vi "EOL Audit Display Data.vi"(7 "Check Position":T2, 8 "Check Noise Test":T2, 9 "Audit Motion Database Table":T3={"Motion"=enum."Glass Teach", "Actual Avg Current"=0.0, "Actual Runtime"=0.0, "Actual Speed"=0.0, "Current Data"=[], "Motion Data Limits"={"Power Supply Voltage"=0.0, "Min Avg Current"=0.0, "Max Avg Current"=0.0, "Min Run Time"=0.0, "Max Run Time"=0.0, "Min Speed"=0.0, "Max Speed"=0.0, "AP Data % of Threshold"=10.0, "Travel Distance"=0.0, "AP Data Type"=enum."91/61", "Check Current"=FALSE, "Check Run Time"=FALSE, "Check Speed"=FALSE, "Express Motion?"=FALSE, "Check Sound Test"=FALSE, "Check Position?"=FALSE, "Collect AP Data"=FALSE, "Inital Position"=0, "End Position"=0, "Goto Posiition"=0, "Max max Current"=0.0, "Min max Current"=0.0, "Check max Current"=FALSE, "Check Sound"=FALSE, "Min Sound (dB)"=0.0, "Max Sound (dB)"=0.0, "SW Mode"=enum."Hard Switch", "LIN Msg"={"ID"=0, "Msg"=[], "LDF"="EX1H"}}, "Switch 1 to 6"=[], "Actual PS Voltage"=0.0, "AP Data"=[], "Actual max Current"=0.0, "Actual Noise (dB)"=0.0} {"Motion Data Limits"."LIN Msg"."Msg" format="%02x"; "Motion Data Limits"."LIN Msg"."ID" format="%02x"}) -> (2 "Limits Data":T1 {"Speed" format="%.2g"; "Run Time" format="%.2g"; "Avg Current" format="%.2g"}, 3 "Actual Data":T1 {"Speed" format="%.2g"; "Run Time" format="%.2g"; "Avg Current" format="%.2g"})   [LabVIEW 2018]
uses:
  02.Type Def's/EOL Motion Database Table.ctl
  02.Type Def's/All Motions.ctl
  05.UserVI's/type defs/17x Audit Motion Data Seq Control.ctl
  05.UserVI's/type defs/17x AP Data Type.ctl
  02.Type Def's/Pass Fail Control.ctl
  02.Type Def's/Screen Motion Data.ctl
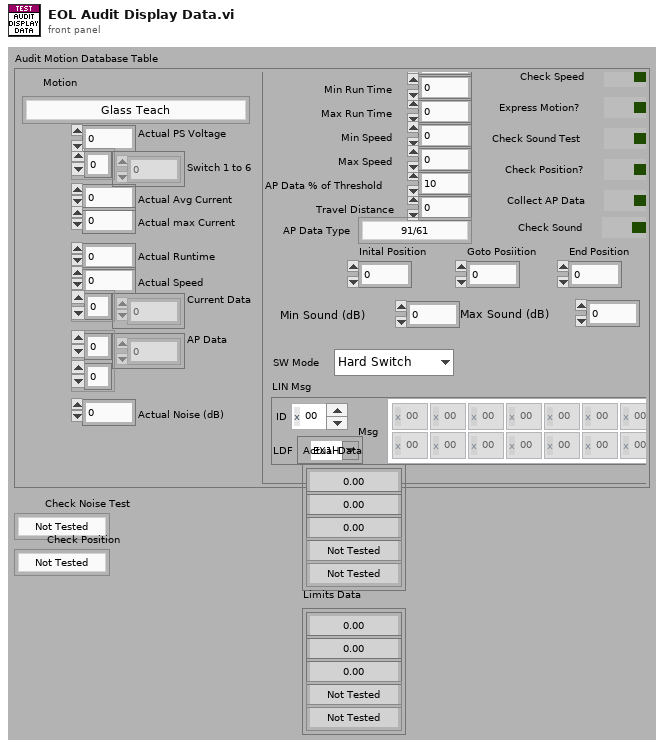
[diagram p1: front panel]
types:
  T1 = typedef "Screen Motion Data.ctl" = cluster{"Noise Test":T2, "Avg Current":dbl, "Run Time":dbl, "Speed":dbl, "Position":T2}
  T2 = typedef "Pass Fail Control.ctl" = enum16{"Not Tested", "Pass", "Fail"}
  T3 = typedef "EOL Motion Database Table.ctl" = cluster{"Motion":T4, "Actual Avg Current":dbl, "Actual Runtime":dbl, "Actual Speed":dbl, "Current Data":sgl[], "Motion Data Limits":T5, "Switch 1 to 6":dbl[], "Actual PS Voltage":dbl, "AP Data":i16[][], "Actual max Current":dbl, "Actual Noise (dB)":dbl}
  T4 = typedef "All Motions.ctl" = enum16{"Glass Teach", "Glass Slide Open", "Glass Slide Close", "Glass Vent Open", "Glass Vent Close", "Sunshade Teach", "Sunshade Open", "Sunshade Close", "Idle", "Sunshade Open 2", "Sunshade Close 2", "Glass Slide Open Sunshade Open", "Glass Slide Open Sunshade Close", "Glass Slide Close Sunshade Open", "Glass Slide Close Sunshade Close", "Glass Vent Open Sunshade Open", "Glass Vent Open Sunshade Close", "Glass Vent Close Sunshade Open", "Glass Vent Close Sunshade Close", "Express Glass Slide Open", "Express Glass Slide Close", "Express Glass Vent Open", "Express Glass Vent Close", "Express Sunshade Open", "Express Sunshade Close", "Express Sunshade Open 2", "Express Sunshade Close 2", "Express Glass Slide Open Sunshade Open", "Express Glass Slide Open Sunshade Close", "Express Glass Slide Close Sunshade Open", "Express Glass Slide Close Sunshade Close", "Express Glass Vent Open Sunshade Open", "Express Glass Vent Open Sunshade Close", "Express Glass Vent Close Sunshade Open", "Express Glass Vent Close Sunshade Close", "Goto Position Glass", "Goto Position Sunshade", "Sunshade Teach 2"}
  T5 = typedef "17x Audit Motion Data Seq Control.ctl" = cluster{"Power Supply Voltage":dbl, "Min Avg Current":dbl, "Max Avg Current":dbl, "Min Run Time":dbl, "Max Run Time":dbl, "Min Speed":dbl, "Max Speed":dbl, "AP Data % of Threshold":dbl, "Travel Distance":dbl, "AP Data Type":T6, "Check Current":bool, "Check Run Time":bool, "Check Speed":bool, "Express Motion?":bool, "Check Sound Test":bool, "Check Position?":bool, "Collect AP Data":bool, "Inital Position":u16, "End Position":u16, "Goto Posiition":u16, "Max max Current":dbl, "Min max Current":dbl, "Check max Current":bool, "Check Sound":bool, "Min Sound (dB)":dbl, "Max Sound (dB)":dbl, "SW Mode":enum16{"Hard Switch", "Uncond Frame"}, "LIN Msg":cluster{"ID":u8, "Msg":u8[][], "LDF":refnum<k21>}}
  T6 = typedef "17x AP Data Type.ctl" = enum16{"91/61", "92/62", "93/63", "67", "68", "6F", "71", "91 Msg", "92 Msg", "93 Msg", "94 Msg", "HiRain 91", "HiRain 92 Speed", "HiRain 92 HS", "HiRain 92", "HiRain 93", "SnT"}
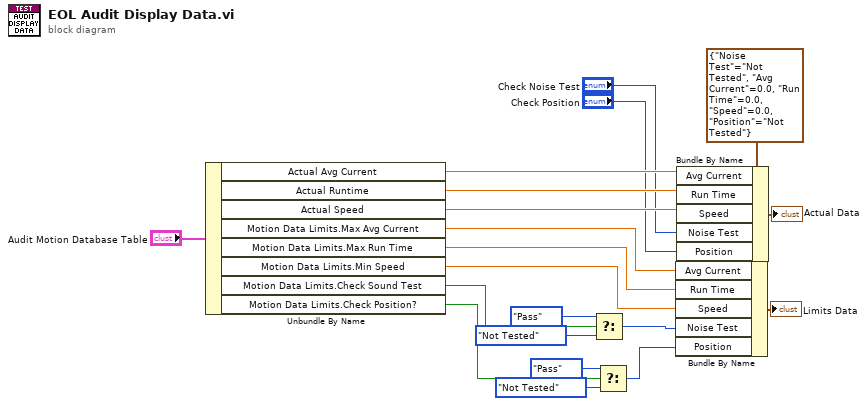
[diagram p0: block diagram]
diagram:
  w9 = T1 {"Noise Test"=enum."Not Tested", "Avg Current"=0.0, "Run Time"=0.0, "Speed"=0.0, "Position"=enum."Not Tested"} ("Slide Open Data")
  n1 = Unbundle By Name("Audit Motion Database Table") -> ("Actual Avg Current"=w6:dbl, "Actual Runtime"=w7:dbl, "Actual Speed"=w8:dbl, "Motion Data Limits.Max Avg Current"=w10:dbl, "Motion Data Limits.Max Run Time"=w11:dbl, "Motion Data Limits.Min Speed"=w12:dbl, "Motion Data Limits.Check Sound Test"=w13:bool, "Motion Data Limits.Check Position?"=w20:bool)
  n2 = Select(t=Pass_Fail_Control."Pass" ("Noise Test"), s=w13, f=Pass_Fail_Control."Not Tested" ("Noise Test")) -> (s? t:f=w16:T2)
  n3 = Select(t=Pass_Fail_Control."Pass" ("Noise Test"), s=w20, f=Pass_Fail_Control."Not Tested" ("Noise Test")) -> (s? t:f=w19:T2)
  n4 = Bundle By Name(cluster=w9, "Avg Current"=w10, "Run Time"=w11, "Speed"=w12, "Noise Test"=w16, "Position"=w19) -> (→"Limits Data":T1)
  n5 = Bundle By Name(cluster=w9, "Avg Current"=w6, "Run Time"=w7, "Speed"=w8, "Noise Test"="Check Noise Test", "Position"="Check Position") -> (→"Actual Data":T1)
